vi "Lens Driver.vi"(8 "error in (no error)":errorcluster, 10 "remote":bool, 11 "VISA resource name":refnum<visa-resource-name>="COM5") -> (0 "error out":errorcluster)   [LabVIEW 2013]
doc: "This VI provides a GUI to control the Optotune Lens Driver. It can be called by a parallel running VI which sends the current values using global variables (Global Lens Driver.vi)."
uses:
  03 Type Def & Global/Slider.ctl
  03 Type Def & Global/Slider Freq.ctl
  03 Type Def & Global/Slider Focal Power.ctl
  03 Type Def & Global/Slider Temperature.ctl
  03 Type Def & Global/Calibration.ctl
  <vilib>/Utility/miscctls.llb/LVPointTypeDef.ctl
  <vilib>/Instr/_visa.llb/VISA Configure Serial Port (Instr).vi
panel:
  out "ID":u16
  in  "Signal B":u16(ring) items=["DC", "Sinus", "Square", "Triangle"]
  in  "Current":T5={"Current dc A"=0.0, "Current dc B"=0.0, "Frequency A"=0.0, "Frequency B"=0.0, "Current hi A"=0.0, "Current hi B"=0.0, "Current low A"=0.0, "Current low B"=0.0, "Focal Power A"=2.0, "Temperature low A"=45.0, "Temperature high A"=20.0} {"Temperature high A" scale=10.0..100.0; "Temperature low A" scale=10.0..100.0; "Focal Power A" scale=-5.0..10.0 scale format="%#_5g"; "Current hi B" scale=-200.0..200.0 scale format="%#_5g"; "Current hi A" scale=-200.0..200.0 scale format="%#_5g"; "Current low B" scale=-200.0..200.0 scale format="%#_5g"; "Current low A" scale=-200.0..200.0 scale format="%#_5g"; "Current dc B" scale=-200.0..200.0 scale format="%#_5g"; "Current dc A" scale=-200.0..200.0 scale format="%#_5g"; "Frequency B" scale=0.1..1000.0; "Frequency A" scale=0.1..1000.0}
  in  "Signal A":u16(ring) items=["DC", "Sinus", "Square", "Triangle", "Focal Power"]
  out "Calibration 2":T6 {"Max Current A" format="%#_g mA"; "Max Current B" format="%#_g mA"; "UCL A" format="%#_g mA"; "LCL A" format="%#_g mA"; "UCL B" format="%#_g mA"; "LCL B" format="%#_g mA"}
  in  "Set Calibration":bool
  out "Data Log":string
  in  "Back":bool
  in  "Command":bool
  in  "command":string
  in  "End VI":bool
  in  "Reset":bool
  in  "Fast":bool
  in  "Temp":bool
  out "Temperature B":dbl format="%#_g °C"
  out "Temperature A":dbl format="%#_g °C"
  out "OK":bool
  out "Data":string
  # "Optotune Lens Driver"
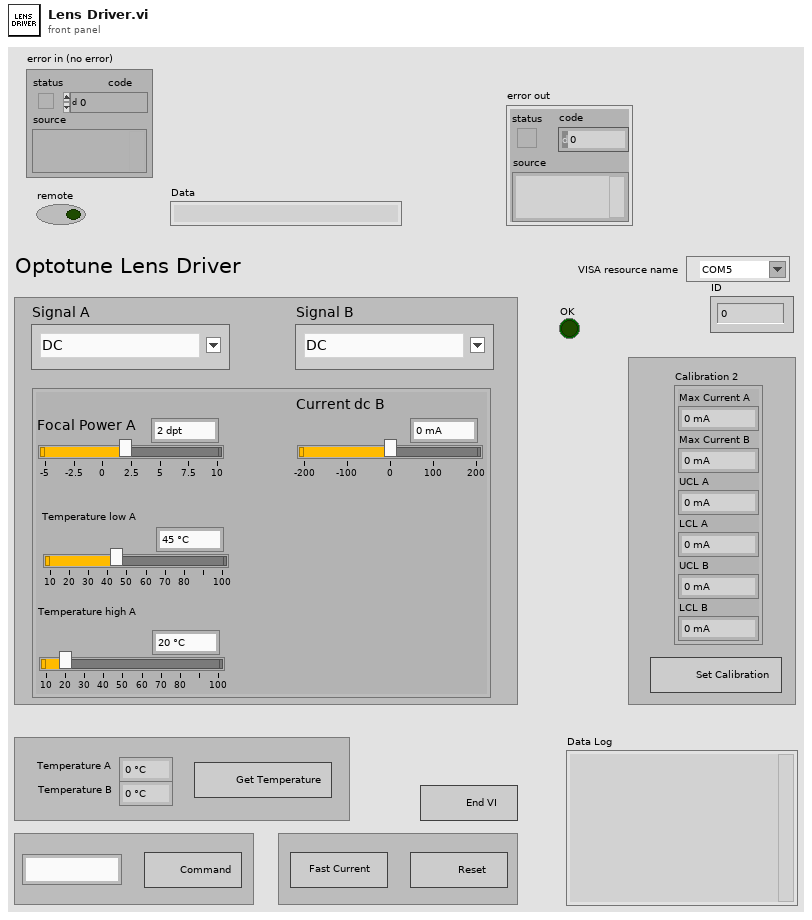
[diagram p1: front panel]
types:
  T1 = typedef "Slider.ctl" = dbl
  T2 = typedef "Slider Freq.ctl" = dbl
  T3 = typedef "Slider Focal Power.ctl" = dbl
  T4 = typedef "Slider Temperature.ctl" = dbl
  T5 = cluster{"Current dc A":T1, "Current dc B":T1, "Frequency A":T2, "Frequency B":T2, "Current hi A":T1, "Current hi B":T1, "Current low A":T1, "Current low B":T1, "Focal Power A":T3, "Temperature low A":T4, "Temperature high A":T4}
  T6 = typedef "Calibration.ctl" = cluster{"Max Current A":dbl, "Max Current B":dbl, "UCL A":dbl, "UCL B":dbl, "LCL A":dbl, "LCL B":dbl}
  T7 = typedef "LVPointTypeDef.ctl" = cluster{"Horizontal":i16, "Vertical":i16}
  T8 = cluster{"Current dc A":T1, "Current dc B":T1, "Frequency A":T2, "Frequency B":T2, "Current hi A":T1, "Current hi B":T1, "Current low A":T1, "Current low B":T1, "Focal Power A":T3, "Temperature high A":T4, "Temperature low A":T4}
  T9 = cluster{"Current dc A":bool, "Current dc B":bool, "Frequency A":bool, "Frequency B":bool, "Current hi A":bool, "Current hi B":bool, "Current low A":bool, "Current low B":bool, "Focal Power A":bool, bool, bool}
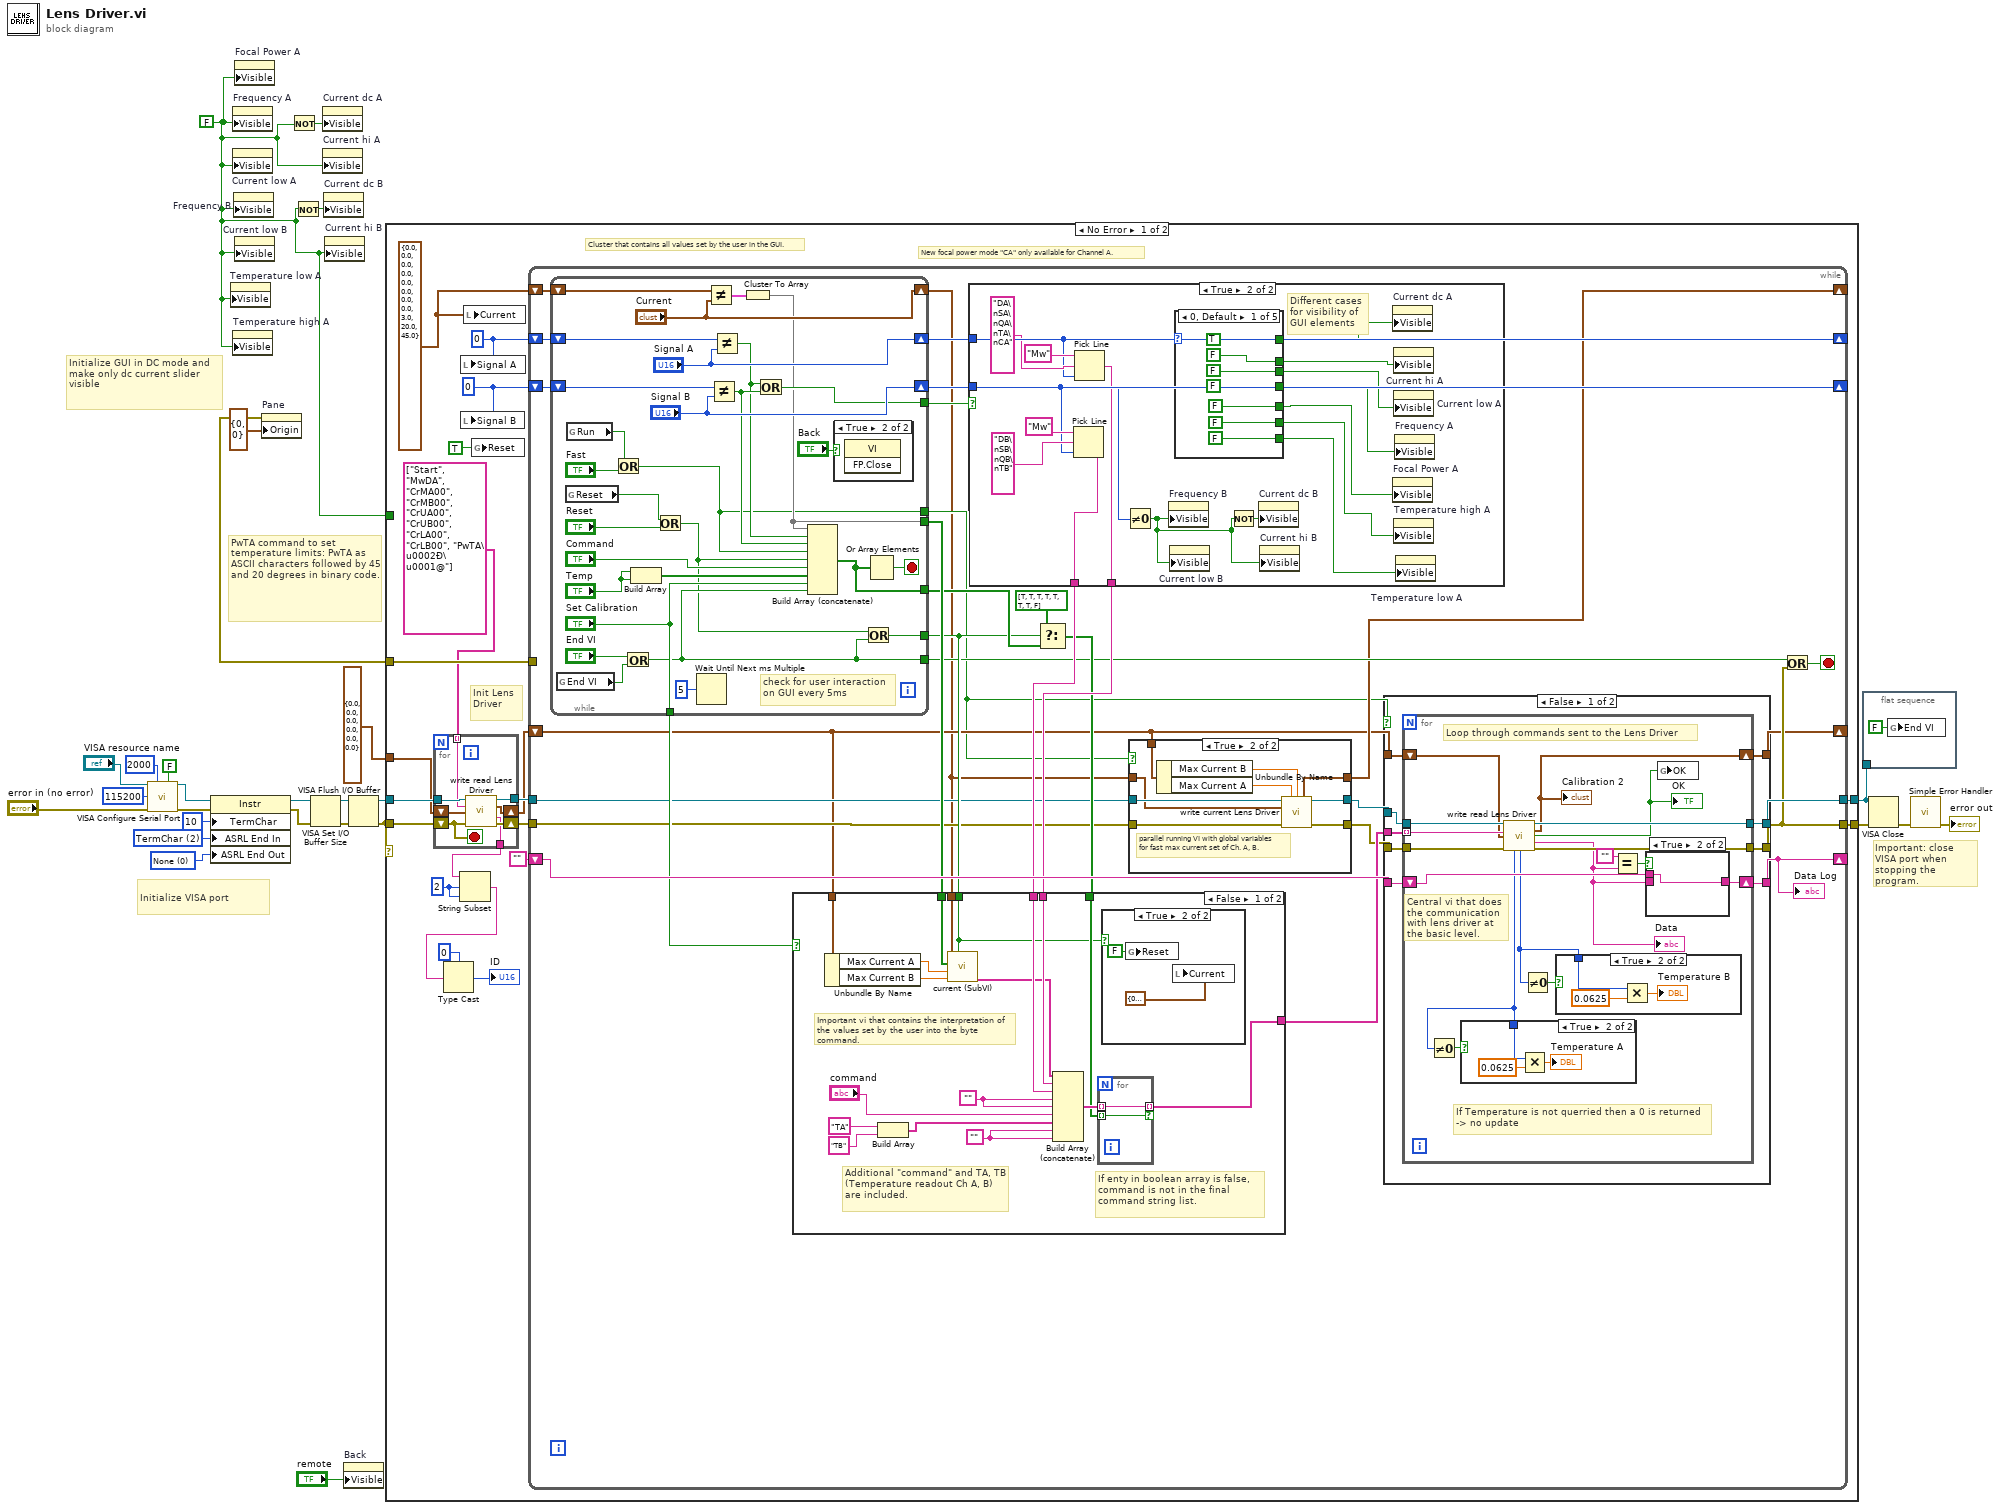
[diagram p0: block diagram]
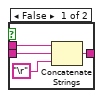
[diagram p4: hidden frame]
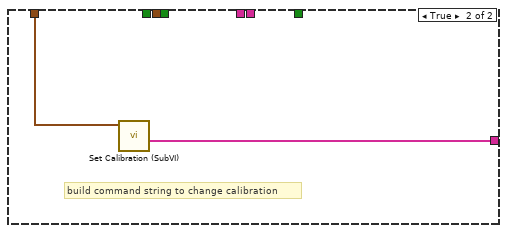
[diagram p8: hidden frame]
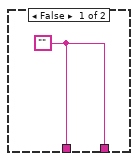
[diagram p9: hidden frame]
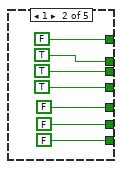
[diagram p10: hidden frame]
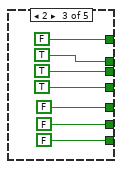
[diagram p11: hidden frame]
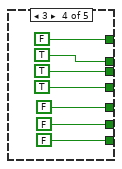
[diagram p12: hidden frame]
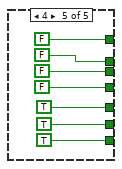
[diagram p13: hidden frame]
diagram:
  w1 = FALSE
  w8 = u16 0 items=["None", "Last Bit", "TermChar", "Break"] ("Serial Settings:End Mode for Writes")
  w9 = u16 2 items=["None", "Last Bit", "TermChar"] ("Serial Settings:End Mode for Reads")
  # "PwTA command to set temperature limits: PwTA as ASCII characters followed by 45 and 20 degrees in binary code."
  # "Important: close VISA port when stopping the program."
  # "Initialize VISA port"
  # "Initialize GUI in DC mode and make only dc current slider visible"
  n1 = call-poly "VISA Configure Serial Port"("VISA resource name"="VISA resource name", "timeout (10sec)"=u32 2000, "Enable Termination\nChar (T)"=FALSE ("Enable Termination\nChar (T)"), "baud rate (9600)"=u32 115200, "error in (no error)"="error in (no error)") -> ("VISA resource name out"=w13:refnum<visa-resource-name>, "error out"=w11:errorcluster)  [unwired: 9 in]
  n2 = property class="Instr"(reference=w13, error in=w11, "TermChar"=u8 10 ("Message Based Settings:Termination Character"), "ASRL End In"=w9, "ASRL End Out"=w8) -> (reference out=w12:refnum<visa-resource-name>, error out=w10:errorcluster)
  n3 = property on="Temperature low A" class="Slide (strict)"("Visible"=w1) -> ()  [unwired: 2 in, 2 out]
  n4 = property on="Frequency A" class="Slide (strict)"("Visible"=w1) -> ()  [unwired: 2 in, 2 out]
  n5 = property on="Current low A" class="Slide (strict)"("Visible"=w1) -> ()  [unwired: 2 in, 2 out]
  n6 = property on="Temperature high A" class="Slide (strict)"("Visible"=w1) -> ()  [unwired: 2 in, 2 out]
  n7 = property on="Frequency B" class="Slide (strict)"("Visible"=w1) -> ()  [unwired: 2 in, 2 out]
  n8 = property on="Focal Power A" class="Slide (strict)"("Visible"=w1) -> ()  [unwired: 2 in, 2 out]
  n9 = property on="Current low B" class="Slide (strict)"("Visible"=w1) -> ()  [unwired: 2 in, 2 out]
  n10 = property on="Pane" class="Pane"("Origin"=T7 {"Horizontal"=0, "Vertical"=0}) -> (error out=w16:errorcluster)  [unwired: 2 in, 1 out]
  n11 = Not(x=w1) -> (.not. x?=w4:bool)
  n12 = Not(x=w1) -> (.not. x?=w5:bool)
  n13 = VISA Set I/O Buffer Size(VISA resource name=w12, error in (no error)=w10) -> (VISA resource name out=w23:refnum<visa-resource-name>, error out=w22:errorcluster)  [unwired: 2 in]
  n14 = property on="Current dc A" class="Slide (strict)"("Visible"=w4) -> ()  [unwired: 2 in, 2 out]
  n15 = property on="Current hi A" class="Slide (strict)"("Visible"=w1) -> ()  [unwired: 2 in, 2 out]
  n16 = property on="Current dc B" class="Slide (strict)"("Visible"=w5) -> ()  [unwired: 2 in, 2 out]
  n17 = property on="Current hi B" class="Slide (strict)"("Visible"=w1) -> ()  [unwired: 2 in, 2 out]
  n18 = property on="Back" class="Bool"("Visible"="remote") -> ()  [unwired: 2 in, 2 out]
  n19 = VISA Flush I/O Buffer(VISA resource name=w23, error in (no error)=w22) -> (VISA resource name out=w19:refnum<visa-resource-name>, error out=w15:errorcluster)  [unwired: 1 in]
  n20 = case shown="No Error" w15 {
    tunnel: [w47 w246] -> w14
    tunnel: [w46 w245] -> w21
    tunnel: w19 -> [w44 w246]
    tunnel: w15 -> [w43 w245]
    tunnel: w16 -> [w40 _]
    tunnel: T6 {"Max Current A"=0.0, "Max Current B"=0.0, "UCL A"=0.0, "UCL B"=0.0, "LCL A"=0.0, "LCL B"=0.0} ("Calibration 3") -> [w30 _]
    tunnel: w1 -> [_ _]
    frame No Error {
      w29 = T8 {"Current dc A"=0.0, "Current dc B"=0.0, "Frequency A"=0.0, "Frequency B"=0.0, "Current hi A"=0.0, "Current hi B"=0.0, "Current low A"=0.0, "Current low B"=0.0, "Focal Power A"=3.0, "Temperature high A"=20.0, "Temperature low A"=45.0} ("Current")
      w36 = 2 ("length (rest)")
      w38 = u16 0 ("Signal B")
      w37 = u16 0 ("Signal A")
      # "New focal power mode \"CA\" only available for Channel A."
      # "Cluster that contains all values set by the user in the GUI."
      # "Init Lens Driver"
      n21 = for {
        tunnel: w44 -> [w55]
        tunnel: [w54] -> w42
        tunnel: string[] ["Start", "MwDA", "CrMA00", "CrMB00", "CrUA00", "CrUB00", "CrLA00", "CrLB00", "PwTA\u0002Ð\u0001@"] -> [w52] mode=indexing
        shift-right: [w53] -> w41
        shift-left: w43 -> [w48]
        shift-right: [w50] -> w39
        shift-left: w30 -> [w51]
        tunnel: [w49] -> w34
        stop <- w48 stop-if-true
        n22 = call "write read Lens Driver.vi"("VISA resource name"=w55, "command"=w52, "Calibration"=w51, "error in (no error)"=w48) -> ("VISA resource name out"=w54:refnum<visa-resource-name>, "Calibration 2"=w50:T6, "Data"=w49:string, "error out"=w53:errorcluster)  [unwired: 4 in, 4 out]
      }
      n23 = String Subset(string=w34, offset (0)=w36, length (rest)=w36) -> (substring=w32:string)
      n24 = Type Cast(type=u16 0 ("length (rest)"), x=w32) -> (*(type *) &x=→"ID":u16)
      n25 = local write "Signal A"(w37) -> ()
      n26 = local write "Signal B"(w38) -> ()
      n27 = local write "Current"(w29) -> ()
      n28 = global write "Global Lens Driver.vi" "Reset"(TRUE ("Reset")) -> ()
      n29 = while {
        tunnel: w42 -> [w61]
        tunnel: [w85] -> w47
        tunnel: [w80] -> w46
        tunnel: w41 -> [w60]
        shift-right: [w84] -> _
        shift-left: "" -> [w83]
        tunnel: w40 -> [_]
        shift-right: [w79] -> _
        shift-left: w39 -> [w58]
        shift-right: [w59] -> _
        shift-left: w29 -> [w66]
        shift-right: [w74] -> _
        shift-left: w37 -> [w73]
        shift-right: [w75] -> _
        shift-left: w38 -> [w76]
        stop <- w81 stop-if-true
        n30 = while {
          tunnel: ["Set Calibration"] -> w82
          tunnel: [w220] -> w64
          tunnel: [w236] -> w68
          shift-right: ["Signal A"] -> w74
          shift-left: w73 -> [w235]
          shift-right: ["Signal B"] -> w75
          shift-left: w76 -> [w233]
          shift-right: ["Current"] -> w56
          shift-left: w66 -> [w231]
          tunnel: [w226] -> w72
          tunnel: [w225] -> w71
          tunnel: [w219] -> w65
          tunnel: [w216] -> w57
          stop <- w237 stop-if-true
          # "check for user interaction\non GUI every 5ms"
          n31 = global read "Global Lens Driver.vi" "End VI"() -> (w222:bool)
          n32 = global read "Global Lens Driver.vi" "Reset"() -> (w241:bool)
          n33 = global read "Global Lens Driver.vi" "Run"() -> (w217:bool)
          n34 = Or(x=w217, y="Fast") -> (x .or. y?=w216:bool)
          n35 = Or(x="End VI", y=w222) -> (x .or. y?=w220:bool)
          n36 = Build Array("Temp", "Temp") -> (w224:bool[])
          n37 = Or(x=w241, y="Reset") -> (x .or. y?=w218:bool)
          n38 = Wait Until Next ms Multiple(millisecond multiple=u32 5) -> ()  [unwired: 1 out]
          n39 = Not Equal?(x=w231, y="Current") -> (x != y?=w229:T9)
          n40 = Not Equal?(x=w233, y="Signal B") -> (x != y?=w228:bool)
          n41 = Not Equal?(x=w235, y="Signal A") -> (x != y?=w227:bool)
          n42 = Cluster To Array(cluster=w229) -> (array=w225:bool[])
          n43 = Or(x=w227, y=w228) -> (x .or. y?=w226:bool)
          n44 = Build Array (concatenate)(w225, w227, w228, w216, w218, "Command", w224, "Set Calibration", w220) -> (w236:bool[])
          n45 = case shown="True" "Back" {
            frame False {
            }
            frame True {
              n46 = invoke class="VI" method="FP.Close"() -> ()  [unwired: 3 in, 3 out]
            }
          }
          n47 = Or(x=w218, y=w220) -> (x .or. y?=w219:bool)
          n48 = Or Array Elements(Boolean array=w236) -> (logical OR=w237:bool)
        }
        n49 = case shown="True" w72 {
          tunnel: [w163 w176] -> w78
          tunnel: [w163 w175] -> w77
          tunnel: w75 -> [_ w174]
          tunnel: w74 -> [_ w171]
          frame False {
            w163 = ""
          }
          frame True {
            # "Different cases for visibility of GUI elements"
            n50 = Pick Line(string ("")="Mw", multi-line string="DB\nSB\nQB\nTB", line index=w174) -> (output string=w175:string)
            n51 = Pick Line(string ("")="Mw", multi-line string="DA\nSA\nQA\nTA\nCA", line index=w171) -> (output string=w176:string)
            n52 = Not Equal To 0?(x=w174) -> (x != 0?=w173:bool)
            n53 = property on="Frequency B" class="Slide (strict)"("Visible"=w173) -> ()  [unwired: 2 in, 2 out]
            n54 = property on="Current low B" class="Slide (strict)"("Visible"=w173) -> ()  [unwired: 2 in, 2 out]
            n55 = case shown="0, Default" w171 {
              tunnel: [TRUE FALSE FALSE FALSE FALSE] -> w170
              tunnel: [FALSE TRUE TRUE TRUE FALSE] -> w169
              tunnel: [FALSE TRUE TRUE TRUE FALSE] -> w168
              tunnel: [FALSE TRUE TRUE TRUE FALSE] -> w167
              tunnel: [FALSE FALSE FALSE FALSE TRUE] -> w166
              tunnel: [FALSE FALSE FALSE FALSE TRUE] -> w165
              tunnel: [FALSE FALSE FALSE FALSE TRUE] -> w164
              frame 0, Default {
              }
              frame 1 {
              }
              frame 2 {
              }
              frame 3 {
              }
              frame 4 {
              }
            }
            n56 = Not(x=w173) -> (.not. x?=w172:bool)
            n57 = property on="Current dc B" class="Slide (strict)"("Visible"=w172) -> ()  [unwired: 2 in, 2 out]
            n58 = property on="Current hi B" class="Slide (strict)"("Visible"=w173) -> ()  [unwired: 2 in, 2 out]
            n59 = property on="Current dc A" class="Slide (strict)"("Visible"=w170) -> ()  [unwired: 2 in, 2 out]
            n60 = property on="Focal Power A" class="Slide (strict)"("Visible"=w166) -> ()  [unwired: 2 in, 2 out]
            n61 = property on="Current hi A" class="Slide (strict)"("Visible"=w169) -> ()  [unwired: 2 in, 2 out]
            n62 = property on="Current low A" class="Slide (strict)"("Visible"=w168) -> ()  [unwired: 2 in, 2 out]
            n63 = property on="Temperature high A" class="Slide (strict)"("Visible"=w165) -> ()  [unwired: 2 in, 2 out]
            n64 = property on="Frequency A" class="Slide (strict)"("Visible"=w167) -> ()  [unwired: 2 in, 2 out]
            n65 = property on="Temperature low A" class="Slide (strict)"("Visible"=w164) -> ()  [unwired: 2 in, 2 out]
          }
        }
        n66 = Select(t=bool[] [TRUE, TRUE, TRUE, TRUE, TRUE, TRUE, TRUE, FALSE], s=w65, f=w68) -> (s? t:f=w69:bool[])
        n67 = case shown="False" w82 {
          tunnel: [w151 w161] -> w70
          tunnel: w69 -> [w155 _]
          tunnel: w78 -> [w154 _]
          tunnel: w77 -> [w153 _]
          tunnel: w58 -> [w150 w162]
          tunnel: w56 -> [w139 _]
          tunnel: w71 -> [w149 _]
          tunnel: w65 -> [w140 _]
          frame False {
            w142 = ""
            w152 = ""
            # "Additional \"command\" and TA, TB (Temperature readout Ch A, B) are included."
            # "Important vi that contains the interpretation of the values set by the user into the byte command."
            # "If enty in boolean array is false, command is not in the final command string list."
            n68 = Unbundle By Name(w150) -> ("Max Current A"=w147:dbl, "Max Current B"=w148:dbl)
            n69 = Build Array("TA", "TB") -> (w143:string[])
            n70 = call "current (SubVI).vi"("Reset"=w140, "Max Current B"=w148, "Max Current A"=w147, "Array"=w149, "Current"=w139) -> ("command"=w146:string[])  [unwired: 6 in]
            n71 = Build Array (concatenate)(w146, w154, w153, w142, w142, "command", w143, w152, w152) -> (w156:string[])
            n72 = for {
              tunnel: w156 -> [w160] mode=indexing
              tunnel: w155 -> [w159] mode=indexing
              tunnel: [w160] -> w151 mode=indexing if=w159
            }
            n73 = case shown="True" w140 {
              frame False {
              }
              frame True {
                n74 = global write "Global Lens Driver.vi" "Reset"(FALSE ("Reset")) -> ()
                n75 = local write "Current"(T8 {"Current dc A"=0.0, "Current dc B"=0.0, "Frequency A"=0.0, "Frequency B"=0.0, "Current hi A"=0.0, "Current hi B"=0.0, "Current low A"=0.0, "Current low B"=0.0, "Focal Power A"=0.0, "Temperature high A"=20.0, "Temperature low A"=45.0} ("Current")) -> ()
              }
            }
          }
          frame True {
            # "build command string to change calibration"
            n76 = call "Set Calibration (SubVI).vi"("Calibration in"=w162) -> ("Array"=w161:string[])  [unwired: 10 in]
          }
        }
        n77 = case shown="True" w57 {
          tunnel: [w129 w138] -> w63
          tunnel: [w128 w137] -> w62
          tunnel: w61 -> [w129 w136]
          tunnel: w60 -> [w128 w135]
          tunnel: w56 -> [w127 w131]
          tunnel: [w127 w130] -> w59
          tunnel: w58 -> [_ w134]
          frame False {
          }
          frame True {
            # "parallel running VI with global variables\nfor fast max current set of Ch. A, B."
            n78 = Unbundle By Name(w134) -> ("Max Current B"=w133:dbl, "Max Current A"=w132:dbl)
            n79 = call "write current Lens Driver.vi"("VISA resource name"=w136, "Max Current A"=w132, "Max Current B"=w133, "Current"=w131, "error in (no error)"=w135) -> ("Current 3"=w130:T8, "VISA resource name out"=w138:refnum<visa-resource-name>, "error out"=w137:errorcluster)  [unwired: 7 in, 1 out]
          }
        }
        n80 = case shown="False" w57 {
          tunnel: [w94 w125] -> w85
          tunnel: [w93 w123] -> w84
          tunnel: w83 -> [w92 w123]
          tunnel: [w91 w124] -> w80
          tunnel: [w90 w126] -> w79
          tunnel: w70 -> [w89 _]
          tunnel: w63 -> [w88 w125]
          tunnel: w62 -> [w87 w124]
          tunnel: w58 -> [w86 w126]
          frame False {
            n81 = for {
              tunnel: w88 -> [w111]
              tunnel: [w110] -> w94
              tunnel: [w109] -> w91
              tunnel: w87 -> [w108]
              tunnel: w89 -> [w105] mode=indexing
              shift-right: [w107] -> w93
              shift-left: w92 -> [w106]
              shift-right: [w99] -> w90
              shift-left: w86 -> [w104]
              # "Central vi that does the communication with lens driver at the basic level."
              # "Loop through commands sent to the Lens Driver"
              # "If Temperature is not querried then a 0 is returned\n-> no update"
              n82 = call "write read Lens Driver.vi"("VISA resource name"=w111, "command"=w105, "Calibration"=w104, "error in (no error)"=w108) -> ("VISA resource name out"=w110:refnum<visa-resource-name>, "Calibration 2"=w99:T6, "OK"=w95:bool, "Data"=w97:string, "TA"=w101:u16, "TB"=w103:u16, "error out"=w109:errorcluster)  [unwired: 4 in, 1 out]
              "Data" <- w97
              "OK" <- w95
              "Calibration 2" <- w99
              n83 = Not Equal To 0?(x=w101) -> (x != 0?=w102:bool)
              n84 = case shown="True" w102 {
                tunnel: w101 -> [_ w117]
                frame False {
                }
                frame True {
                  n85 = Multiply(x=w117, y=0.0625) -> (x*y=→"Temperature A":dbl)
                }
              }
              n86 = Not Equal To 0?(x=w103) -> (x != 0?=w100:bool)
              n87 = case shown="True" w100 {
                tunnel: w103 -> [_ w113]
                frame False {
                }
                frame True {
                  n88 = Multiply(x=w113, y=0.0625) -> (x*y=→"Temperature B":dbl)
                }
              }
              n89 = Equal?(x="", y=w97) -> (x = y?=w98:bool)
              n90 = case shown="True" w98 {
                tunnel: [w120 w122] -> w107
                tunnel: w106 -> [w119 w122]
                tunnel: w97 -> [w118 _]
                frame False {
                  n91 = Concatenate Strings(w119, w118, "\r") -> (w120:string)
                }
                frame True {
                }
              }
              n92 = global write "Global Lens Driver.vi" "OK"(w95) -> ()
            }
          }
          frame True {
          }
        }
        "Data Log" <- w84
        n93 = Or(x=w64, y=w80) -> (x .or. y?=w81:bool)
      }
    }
    frame Error {
    }
  }
  n94 = flat-sequence {
    tunnel: w14 -> [_]
    frame #0 {
      n95 = global write "Global Lens Driver.vi" "End VI"(FALSE ("End VI")) -> ()
    }
  }
  n96 = VISA Close(VISA resource name=w14, error in (no error)=w21) -> (error out=w25:errorcluster)
  n97 = call <vilib>:"Simple Error Handler.vi"("error in (no error)"=w25) -> ("error out"=→"error out":errorcluster)  [unwired: 4 in, 4 out]
